vi "Destroy Job.vi"(8 "error in (no error)":errorcluster, 11 "Job in":refnum<class "Job.lvclass">) -> (0 "error out":errorcluster, 3 "Job out":refnum<class "Job.lvclass">)   [LabVIEW 2013, in "openCronJob.lvlib" / "Job.lvclass"]
uses:
  Job.lvclass
  Job.lvclass/Job.ctl
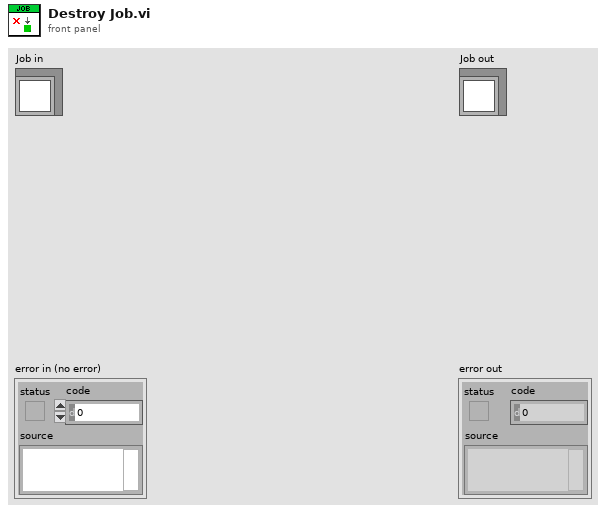
[diagram p1: front panel]
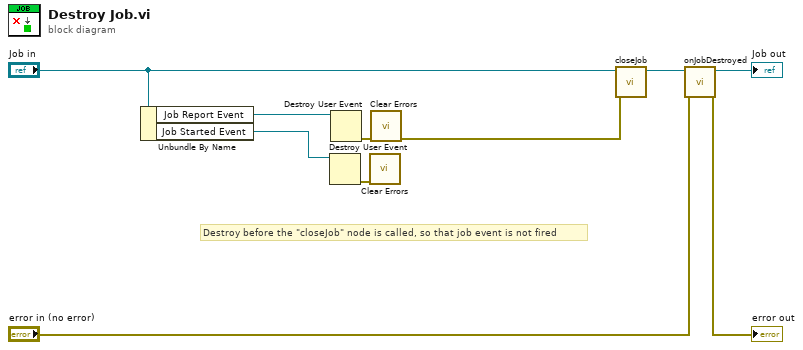
[diagram p0: block diagram]
diagram:
  # "Destroy before the \"closeJob\" node is called, so that job event is not fired"
  n1 = Unbundle By Name("Job in") -> ("Job Report Event"=w10:refnum<user-event>, "Job Started Event"=w1:refnum<user-event>)
  n2 = Destroy User Event(user event=w1) -> (error out=w2:errorcluster)  [unwired: 1 in]
  n3 = Destroy User Event(user event=w10) -> (error out=w9:errorcluster)  [unwired: 1 in]
  n4 = call <vilib>:"Clear Errors.vi"("error in (no error)"=w2) -> ()  [unwired: 6 in, 1 out]
  n5 = call <vilib>:"Clear Errors.vi"("error in (no error)"=w9) -> ("error out"=w7:errorcluster)  [unwired: 6 in]
  n6 = call "closeJob.vi"("error in (no error)"=w7, "Job in"="Job in") -> ("Job out"=w6:refnum<class "Job.lvclass">)  [unwired: 8 in, 1 out]
  n7 = call-dynamic "onJobDestroyed.vi"("error in (no error)"="error in (no error)", "Job in"=w6) -> ("error out"=→"error out":errorcluster, "Job out"=→"Job out":refnum<class "Job.lvclass">)  [unwired: 8 in]
